vi "G_3D.vi"() -> ()   [LabVIEW 2012]
panel:
  out "Ibeomesh":refnum<vi>
  out "Ibeo":refnum<vi>
  out "empty":refnum<vi>
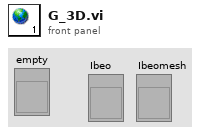
[diagram p1: front panel]
diagram:
